vi "prompt_the_user_but_do_not_linger_v2.0.vi"() -> ()   [LabVIEW 2025]
doc: "Proof of concept/example VI for demonstration.\n\nMichael Panganiban\nSr. Hardware Test Engineer\nFresh Consulting, Inc."
uses:
  controls/home_navigation_btn.ctl
  controls/equipment_navigation_btn.ctl
  controls/settings_navigation_btn.ctl
  controls/test_plan_navigation_btn.ctl
  controls/about_button.ctl
panel:
  in  "about_button":T1
  in  "test_plan":T2
  in  "settings":T3
  in  "equipment":T4
  in  "home":T5
  in  "Tab":T6(tab)
  out "start_of_test_status":string
  in  "start_test":bool
  # "v1.0.0.1"
  # "HOME"
  # "EQUIPMENT"
  # "SETTINGS"
  # "TEST PLAN CREATION"
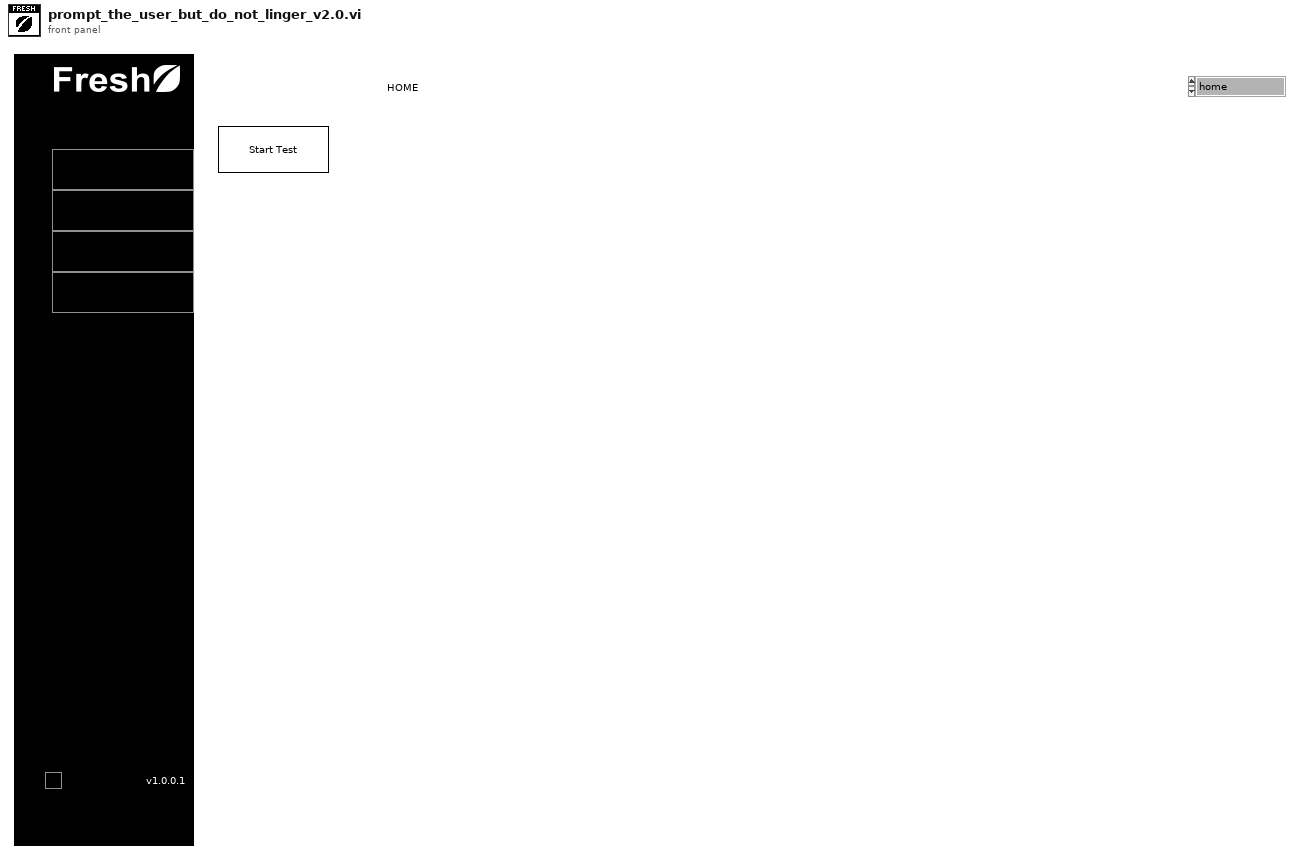
[diagram p1: front panel]
types:
  T1 = typedef "about_button.ctl" = bool
  T2 = typedef "test_plan_navigation_btn.ctl" = bool
  T3 = typedef "settings_navigation_btn.ctl" = bool
  T4 = typedef "equipment_navigation_btn.ctl" = bool
  T5 = typedef "home_navigation_btn.ctl" = bool
  T6 = enum32{"home", "equipment", "settings", "test_plan"}
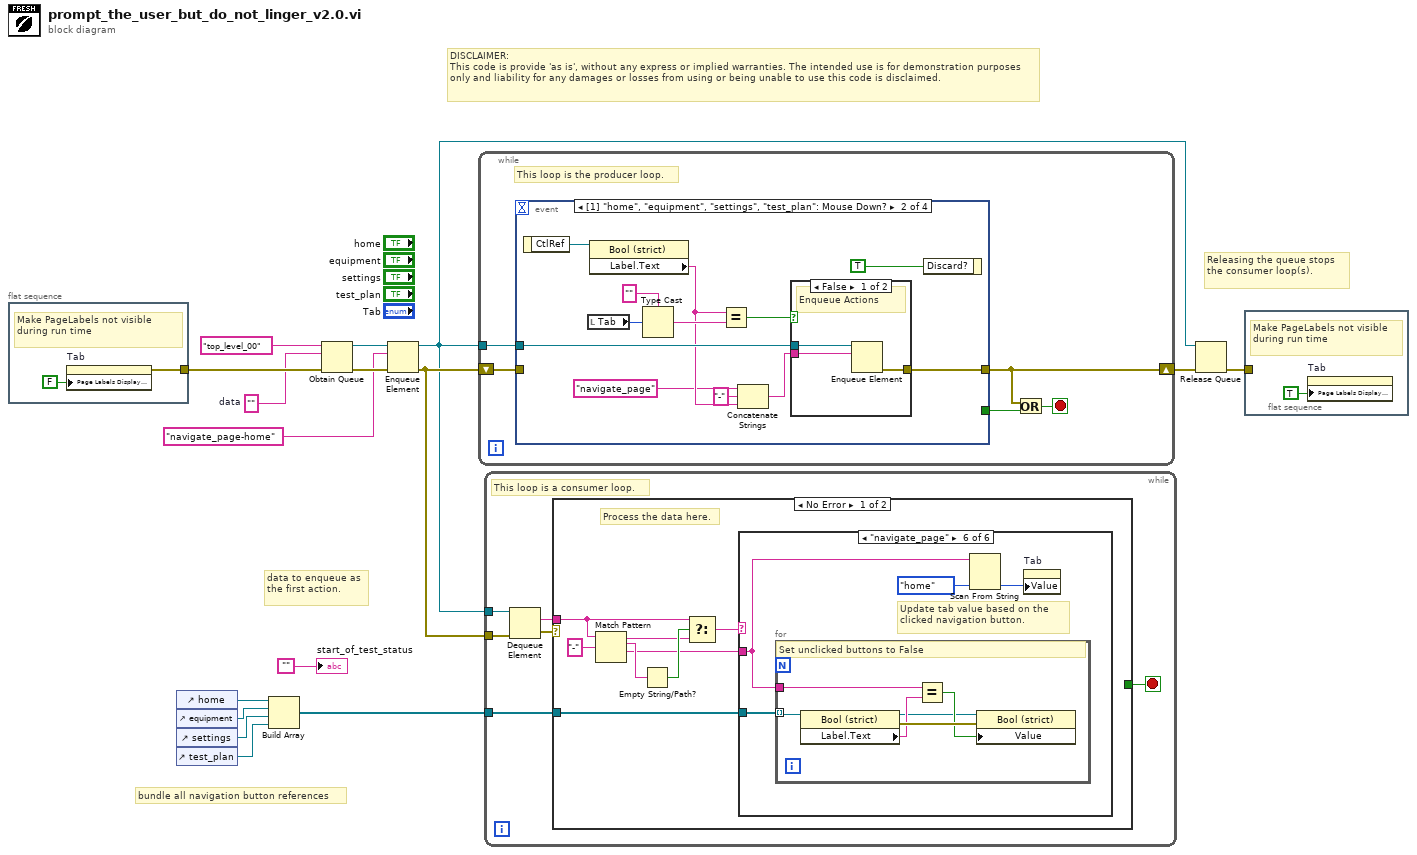
[diagram p0: block diagram]
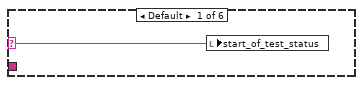
[diagram p2: hidden frame]
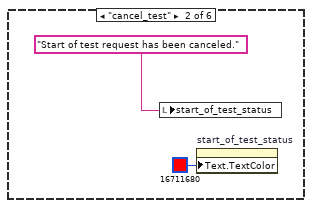
[diagram p3: hidden frame]
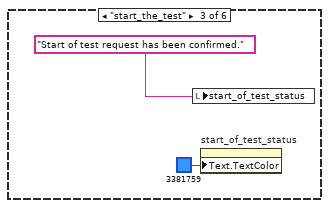
[diagram p4: hidden frame]
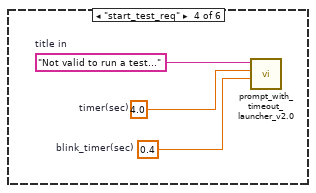
[diagram p5: hidden frame]
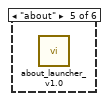
[diagram p6: hidden frame]
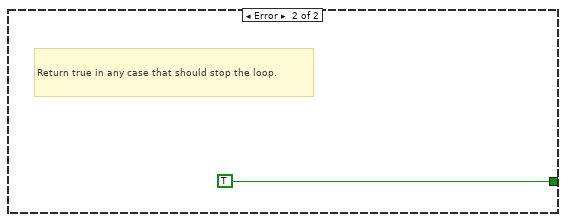
[diagram p7: hidden frame]
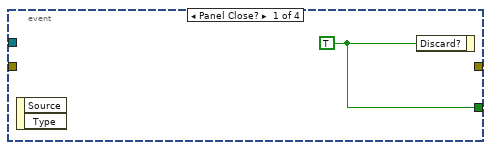
[diagram p8: hidden frame]
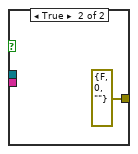
[diagram p9: hidden frame]
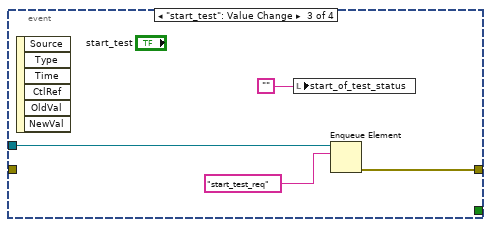
[diagram p10: hidden frame]
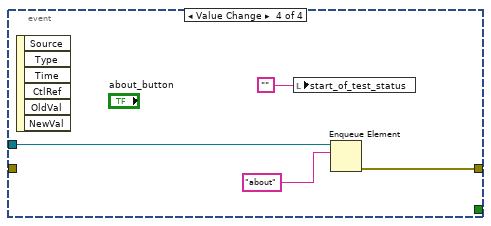
[diagram p11: hidden frame]
diagram:
  w2 = ""  # data
  # "data to enqueue as the first action."
  # "bundle all navigation button references"
  # "DISCLAIMER:\nThis code is provide 'as is', without any express or implied warranties. The intended use is for demonstration purposes only and liability for any damages or losses from using or being unable to use this code is disclaimed."
  # "Releasing the queue stops the consumer loop(s)."
  n1 = flat-sequence {
    tunnel: [w17] -> w15
    frame #0 {
      # "Make PageLabels not visible during run time"
      n2 = property on="Tab" class="TabCtl (strict)"("Page Labels Display Visible?"=FALSE) -> (error out=w17:errorcluster)  [unwired: 2 in, 1 out]
    }
  }
  n3 = control-ref of="home"() -> (w7:refnum<vi>)
  n4 = control-ref of="equipment"() -> (w13:refnum<vi>)
  n5 = control-ref of="settings"() -> (w12:refnum<vi>)
  n6 = control-ref of="test_plan"() -> (w11:refnum<vi>)
  n7 = Build Array(w7, w13, w12, w11) -> (w10:refnum<vi>[])
  n8 = Obtain Queue(name (unnamed)="top_level_00", element data type=w2, error in (no error)=w15) -> (queue out=w9:refnum<queue>, error out=w8:errorcluster)  [unwired: 2 in, 1 out]
  n9 = Enqueue Element(queue=w9, element="navigate_page-home" ("Action"), error in (no error)=w8) -> (queue out=w5:refnum<queue>, error out=w6:errorcluster)  [unwired: 1 in, 1 out]
  n10 = while {
    shift-right: [w20] -> w16
    shift-left: w6 -> [w23]
    tunnel: w5 -> [w19]
    stop <- w21 stop-if-true
    # "This loop is the producer loop."
    n11 = event shown="[1] \"home\", \"equipment\", \"settings\", \"test_plan\": Mouse Down?" {
      selector: _ -> [_ _ _ _]
      dyn-events: _ -> [_ _ _ _]
      timeout: _ -> [_ _ _ _]
      tunnel: w19 -> [_ w35 w44 w48]
      tunnel: w23 -> [_ _ _ _]
      tunnel: [_ w36 w43 w47] -> w20
      tunnel: [w24 _ _ _] -> w22
      event Panel Close? {
        w24 = TRUE ("Discard?")
        n12 = event-data() -> ()  [unwired: 1 in, 2 out]
        n13 = event-data("Discard?"=w24) -> ()  [unwired: 1 in, 1 out]
      }
      event Mouse Down? {
        n14 = event-data() -> ("CtlRef"=w34:refnum<vi>)  [unwired: 1 in]
        n15 = local read "Tab"() -> (w32:T6)
        n16 = property class="Bool (strict)"(reference=w34) -> ("Label.Text"=w28:string)  [unwired: 1 in, 2 out]
        n17 = Type Cast(type="", x=w32) -> (*(type *) &x=w30:string)
        n18 = Equal?(x=w28, y=w30) -> (x = y?=w29:bool)
        n19 = Concatenate Strings("navigate_page" ("string"), "-" ("string"), w28) -> (w25:string)
        n20 = case shown="False" w29 {
          tunnel: [w39 errorcluster {"status"=FALSE, "code"=0, "source"=""} ("error out")] -> w36
          tunnel: w35 -> [w38 _]
          tunnel: w25 -> [w37 _]
          frame False {
            # "Enqueue Actions"
            n21 = Enqueue Element(queue=w38, element=w37) -> (error out=w39:errorcluster)  [unwired: 2 in, 2 out]
          }
          frame True {
          }
        }
        n22 = event-data("Discard?"=TRUE) -> ()  [unwired: 1 in, 1 out]
      }
      event "start_test": Value Change {
        n23 = event-data() -> ()  [unwired: 1 in, 6 out]
        n24 = local write "start_of_test_status"("") -> ()
        n25 = Enqueue Element(queue=w44, element="start_test_req" ("Action")) -> (error out=w43:errorcluster)  [unwired: 2 in, 2 out]
      }
      event Value Change {
        n26 = event-data() -> ()  [unwired: 1 in, 6 out]
        n27 = local write "start_of_test_status"("") -> ()
        n28 = Enqueue Element(queue=w48, element="about" ("Action")) -> (error out=w47:errorcluster)  [unwired: 2 in, 2 out]
      }
    }
    n29 = Or(x=w20, y=w22) -> (x .or. y?=w21:bool)
  }
  n30 = while {
    tunnel: w5 -> [w54]
    tunnel: w10 -> [w50]
    tunnel: w6 -> [w49]
    stop <- w51 stop-if-true
    # "This loop is a consumer loop."
    n31 = Dequeue Element(queue=w54, error in (no error)=w49) -> (element=w52:string, error out=w53:errorcluster)  [unwired: 1 in, 2 out]
    n32 = case shown="No Error" w53 {
      tunnel: w52 -> [w58 _]
      tunnel: [_ TRUE] -> w51
      tunnel: w50 -> [w62 _]
      frame No Error {
        # "Process the data here."
        n33 = Match Pattern(string=w58, regular expression="-") -> (before substring=w57:string, match substring=w60:string, after substring=w55:string)  [unwired: 1 in, 1 out]
        n34 = Empty String/Path?(string/path=w60) -> (empty?=w59:bool)
        n35 = Select(t=w58, s=w59, f=w57) -> (s? t:f=w56:string)
        n36 = case shown="\"navigate_page\"" w56 {
          selector: w56 -> [w63 _ _ _ _ _]
          tunnel: w62 -> [_ _ _ _ _ w72]
          tunnel: w55 -> [_ _ _ _ _ w71]
          frame Default {
            n37 = local write "start_of_test_status"(w63) -> ()
          }
          frame "cancel_test" {
            n38 = local write "start_of_test_status"("Start of test request has been canceled.") -> ()
            n39 = property on="start_of_test_status" class="Str"("Text.TextColor"=u32 16711680 ("Text.Text Colors:Text Color")) -> ()  [unwired: 2 in, 2 out]
          }
          frame "start_the_test" {
            n40 = local write "start_of_test_status"("Start of test request has been confirmed.") -> ()
            n41 = property on="start_of_test_status" class="Str"("Text.TextColor"=u32 3381759 ("Text.Text Colors:Text Color")) -> ()  [unwired: 2 in, 2 out]
          }
          frame "start_test_req" {
            w68 = 0.4  # blink_timer(sec)
            w69 = 4.0  # timer(sec)
            w70 = "Not valid to run a test..."  # title in
            n42 = call "prompt_with_timeout_launcher_v2.0.vi"("blink_timer(sec)"=w68, "timer(sec)"=w69, "message in"=w70) -> ()  [unwired: 8 in, 1 out]
          }
          frame "about" {
            n43 = call "about_launcher_v1.0.vi"() -> ()  [unwired: 11 in, 1 out]
          }
          frame "navigate_page" {
            # "Update tab value based on the clicked navigation button."
            n44 = for {
              tunnel: w72 -> [w80] mode=indexing
              tunnel: w71 -> [w77]
              # "Set unclicked buttons to False"
              n45 = property class="Bool (strict)"(reference=w80) -> (reference out=w75:refnum<vi>, error out=w79:errorcluster, "Label.Text"=w78:string)  [unwired: 1 in]
              n46 = Equal?(x=w77, y=w78) -> (x = y?=w76:bool)
              n47 = property class="Bool (strict)"(reference=w75, error in=w79, "Value"=w76) -> ()  [unwired: 2 out]
            }
            n48 = Scan From String(input string=w71, default 1=T6."home" ("Tab Control")) -> (output 1=w73:T6)  [unwired: 3 in, 3 out]
            n49 = property on="Tab" class="TabCtl (strict)"("Value"=w73) -> ()  [unwired: 2 in, 2 out]
          }
        }
      }
      frame Error {
        # "Return true in any case that should stop the loop."
      }
    }
  }
  n50 = Release Queue(queue=w5, error in (no error)=w16) -> (error out=w14:errorcluster)  [unwired: 1 in, 2 out]
  n51 = flat-sequence {
    tunnel: w14 -> [_]
    frame #0 {
      # "Make PageLabels not visible during run time"
      n52 = property on="Tab" class="TabCtl (strict)"("Page Labels Display Visible?"=TRUE) -> ()  [unwired: 2 in, 2 out]
    }
  }
  "start_of_test_status" <- ""
